vi "putPiece(picture).vi"(6 "drawRed":bool, 8 "posy":i32, 9 "posx":i32, 10 "picture size":dbl, 11 "2D Picture 2":picture) -> (3 "2D Picture":picture)   [LabVIEW 2022 SP3, in "drawPlate.lvlib"]
uses:
  drawPlate.lvlib
panel:
  # "根據輸入的圖片大小、座標和顏色(T黑/F白)畫下一個圓"
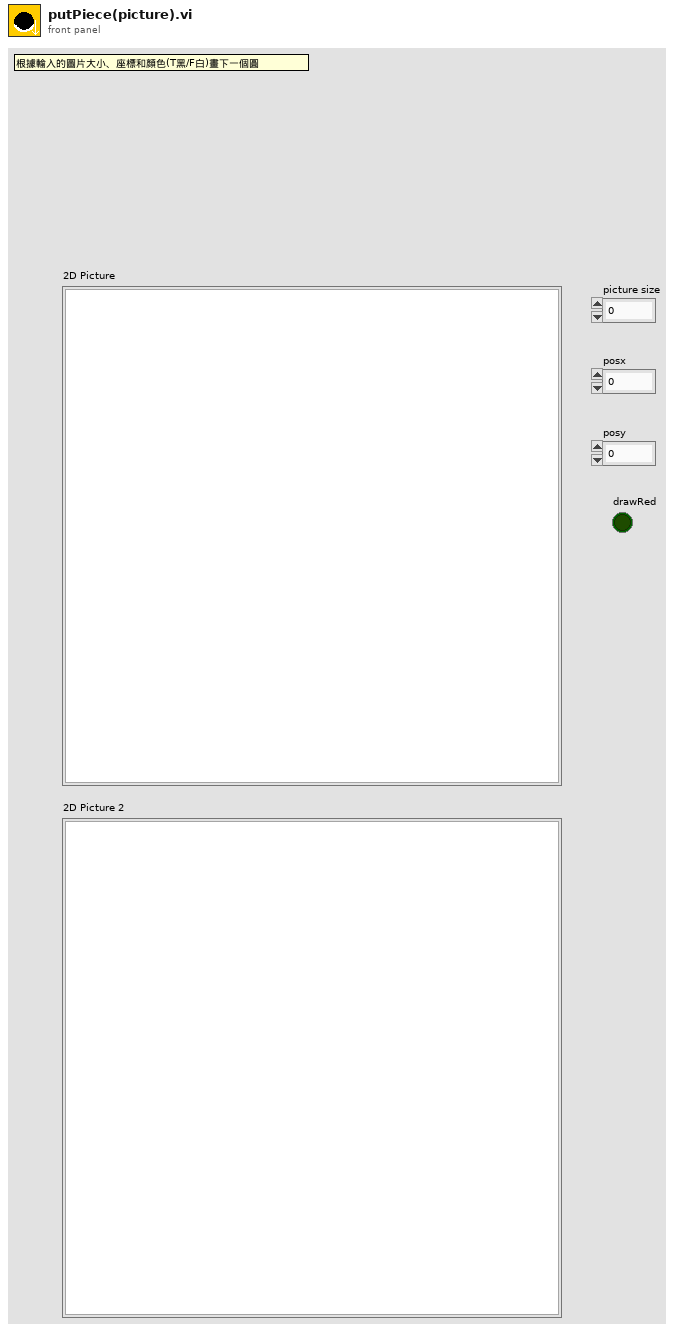
[diagram p1: front panel]
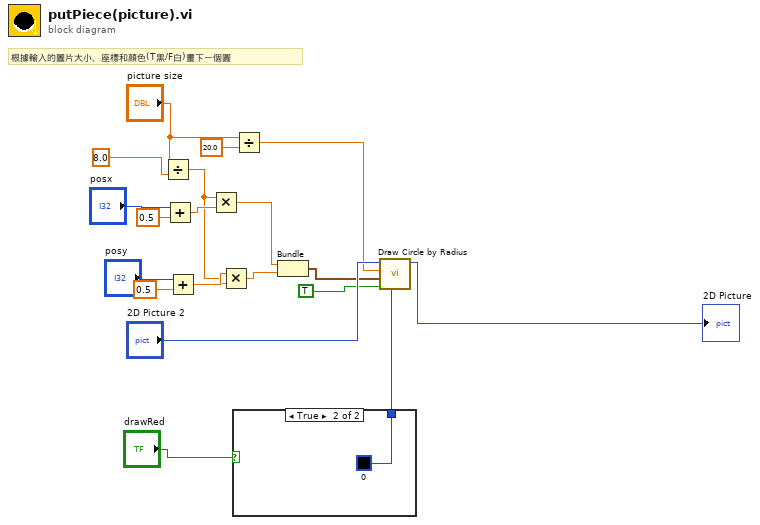
[diagram p0: block diagram]
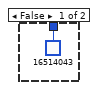
[diagram p2: hidden frame]
diagram:
  # "根據輸入的圖片大小、座標和顏色(T黑/F白)畫下一個圓"
  n1 = Divide(x="picture size", y=8.0) -> (x/y=w5:dbl)
  n2 = Add(x="posx", y=0.5) -> (x+y=w11:dbl)
  n3 = Add(x="posy", y=0.5) -> (x+y=w6:dbl)
  n4 = Multiply(x=w5, y=w11) -> (x*y=w3:dbl)
  n5 = Multiply(x=w6, y=w5) -> (x*y=w4:dbl)
  n6 = case shown="True" "drawRed" {
    tunnel: [u32 16514043 ("color(black)") u32 0 ("color(black)")] -> w1
    frame False {
    }
    frame True {
    }
  }
  n7 = Divide(x="picture size", y=20.0) -> (x/y=w17:dbl)
  n8 = Bundle(w3, w4) -> (w15:cluster{dbl, dbl})  [unwired: 1 in]
  n9 = call <vilib>:"Draw Circle by Radius.vi"("color(black)"=w1, "fill?(F)"=TRUE, "pixel center"=w15, "radius"=w17, "picture"="2D Picture 2") -> ("new picture"=→"2D Picture":picture)  [unwired: 6 in]
